vi "Compiled.Get Counter And Protection Frames.vi"(8 "error in (no error)":errorcluster, 9 "Frames per type":T10[](array[typedef]) {"Frame Settings"."Transmit Trigger Ref" format="%.0x"; "Frame Settings"."Disable Transmission Ref" format="%.0x"; "Frame Refs" format="%.0x"}, 10 "GUIDs":T9, 11 "XNET Cluster":refnum<k21>) -> (0 "error out":errorcluster, 1 "Counters and Protection Refs":T1[](array[typedef]) format="%.0x", 2 "Signals Refs":T1[](array[typedef]) format="%.0x", 3 "Frames":T2[](array[typedef]) {"Protection Configurations"."CRC Channels"."Data Type" items=["Signed", "Unsigned", "IEEE Float"]})   [LabVIEW 2015, in "Protection and Counter Support System Explorer.lvlib"]
uses:
  Protection and Counter Support System Explorer.lvlib
  Types/Export Frames List and Type.ctl
  Shared/Types/Exported Frame Type.ctl
  <vilib>/NI Veristand/Custom Device API/Custom Device Item Ref.ctl
  Types/Exported Frame Settings.ctl
  Shared/Types/Exported Event Trigger Type.ctl
  Types/Export Frame GUIDs List.ctl
  Shared/Types/Exported Frame Settings.ctl
  Shared/Types/Exported Protection Settings.ctl
  Shared/Types/Protection Type.ctl
  Shared/Types/XNET Signal Configuration.ctl
  Shared/Types/Exported Counter Settings.ctl
  <vilib>/NI Veristand/Custom Device Tools/Custom Device Utility Library/NI VeriStand - Search for All Items by GUID.vi
  Shared/Protection and Counter Support Shared.lvlib
  <vilib>/NI VeriStand/Custom Device API/Custom Device API.lvlib
  <resource>/objmgr/xnet.rc
  <vilib>/NI VeriStand/Custom Device Tools/Custom Device Utility Library/Custom Device Utility Library.lvlib
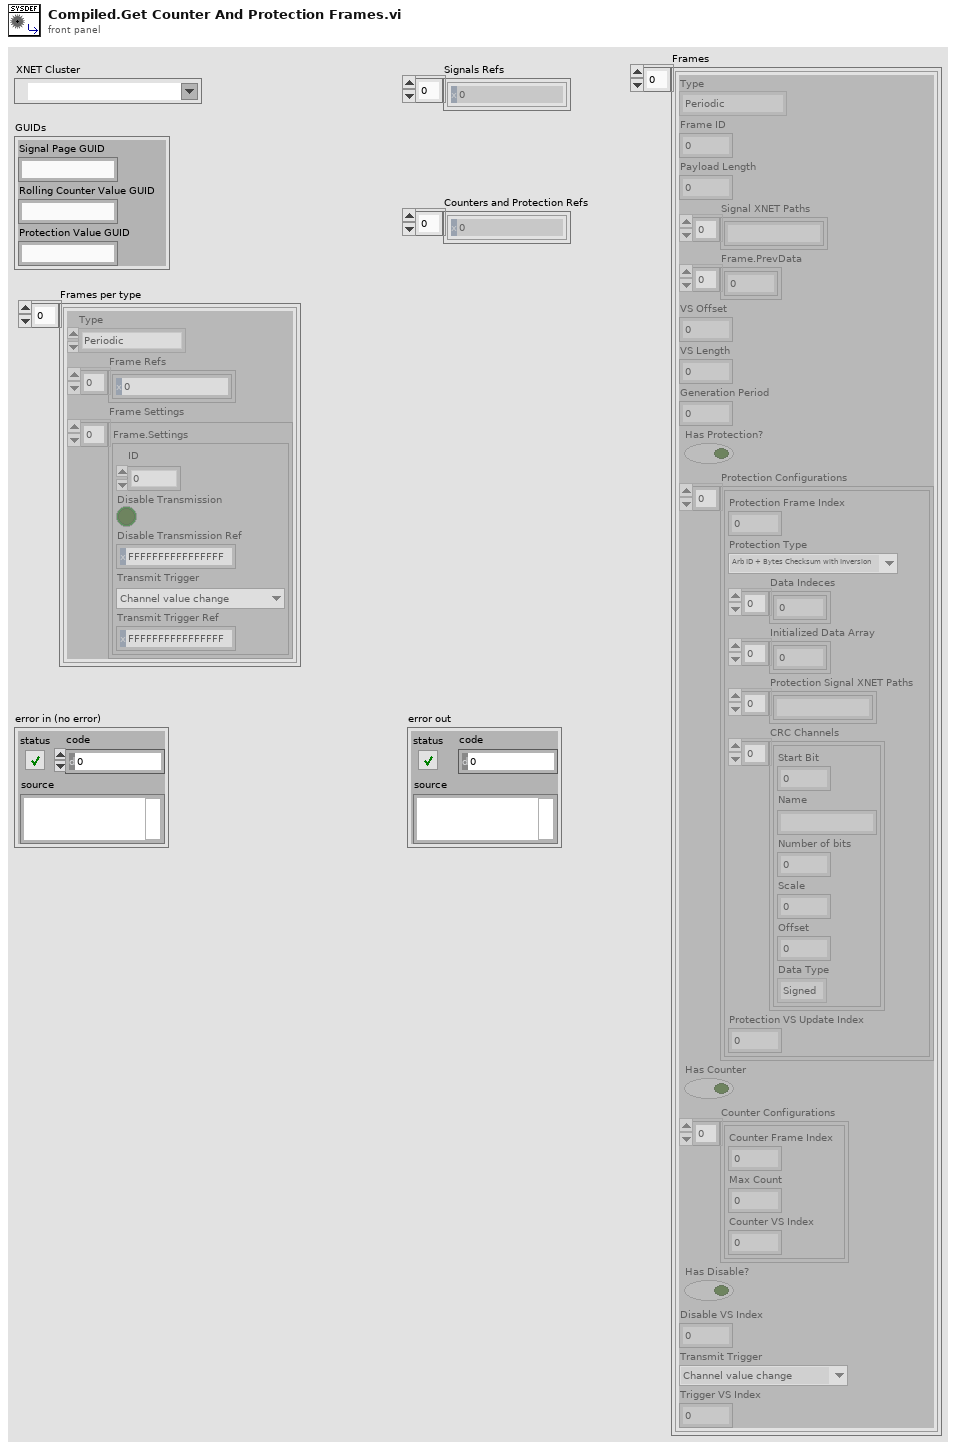
[diagram p1: front panel]
types:
  T1 = typedef "Custom Device API.lvlib/Custom Device Item Ref.ctl" = u64
  T2 = typedef "Protection and Counter Support Shared.lvlib/Exported Frame Settings.ctl" = cluster{"Type":T3, "Frame ID":u32, "Payload Length":u32, "Signal XNET Paths":string[], "Frame.PrevData":dbl[], "VS Offset":i32, "VS Length":i32, "Generation Period":u32, "Has Protection?":bool, "Protection Configurations":T4[], "Has Counter":bool, "Counter Configurations":T7[], "Has Disable?":bool, "Disable VS Index":i32, "Transmit Trigger":T8, "Trigger VS Index":i32}
  T3 = typedef "Protection and Counter Support Shared.lvlib/Exported Frame Type.ctl" = enum16{"Periodic", "Event", "Periodic/Event"}
  T4 = typedef "Protection and Counter Support Shared.lvlib/Exported Protection Settings.ctl" = cluster{"Protection Frame Index":i32, "Protection Type":T5, "Data Indeces":i32[], "Initialized Data Array":dbl[], "Protection Signal XNET Paths":string[], "CRC Channels":T6[], "Protection VS Update Index":i32}
  T5 = typedef "Protection and Counter Support Shared.lvlib/Protection Type.ctl" = enum16{"Arb ID + Bytes Checksum with Inversion", "Arb ID + Bytes CRC with Inversion", "Reversed Raw Signal Checksum with Inversion"}
  T6 = typedef "Protection and Counter Support Shared.lvlib/XNET Signal Configuration.ctl" = cluster{"Start Bit":i32, "Name":string, "Number of bits":i32, "Scale":dbl, "Offset":dbl, "Data Type":u32}
  T7 = typedef "Protection and Counter Support Shared.lvlib/Exported Counter Settings.ctl" = cluster{"Counter Frame Index":i32, "Max Count":dbl, "Counter VS Index":i32}
  T8 = typedef "Protection and Counter Support Shared.lvlib/Exported Event Trigger Type.ctl" = enum16{"Channel value change", "Trigger channel (not zero)", "Channel value change or trigger channel (not zero)", "Trigger channel (any value change)", "Channel value change or trigger channel (any value change)"}
  T9 = typedef "Protection and Counter Support System Explorer.lvlib/Export Frame GUIDs List.ctl" = cluster{"Signal Page GUID":string, "Rolling Counter Value GUID":string, "Protection Value GUID":string}
  T10 = typedef "Protection and Counter Support System Explorer.lvlib/Export Frames List and Type.ctl" = cluster{"Type":T3, "Frame Refs":T1[], "Frame Settings":T11[]}
  T11 = typedef "Protection and Counter Support System Explorer.lvlib/Exported Frame Settings.ctl" = cluster{"ID":u32, "Disable Transmission":bool, "Disable Transmission Ref":T1, "Transmit Trigger":T8, "Transmit Trigger Ref":T1}
  T12 = typedef "Custom Device API.lvlib/Custom Device Item Info.ctl" = cluster{"Name":string, "Is Channel":bool, "GUID":string, "Is Waveform":bool}
  T13 = typedef "Protection and Counter Support System Explorer.lvlib/Protection Signal Settings.ctl" = cluster{"Input Channels":T14[], "Protection Type":T5}
  T14 = typedef "Protection and Counter Support System Explorer.lvlib/Protection Signal Linked Channel.ctl" = cluster{"Node Ref":T1}
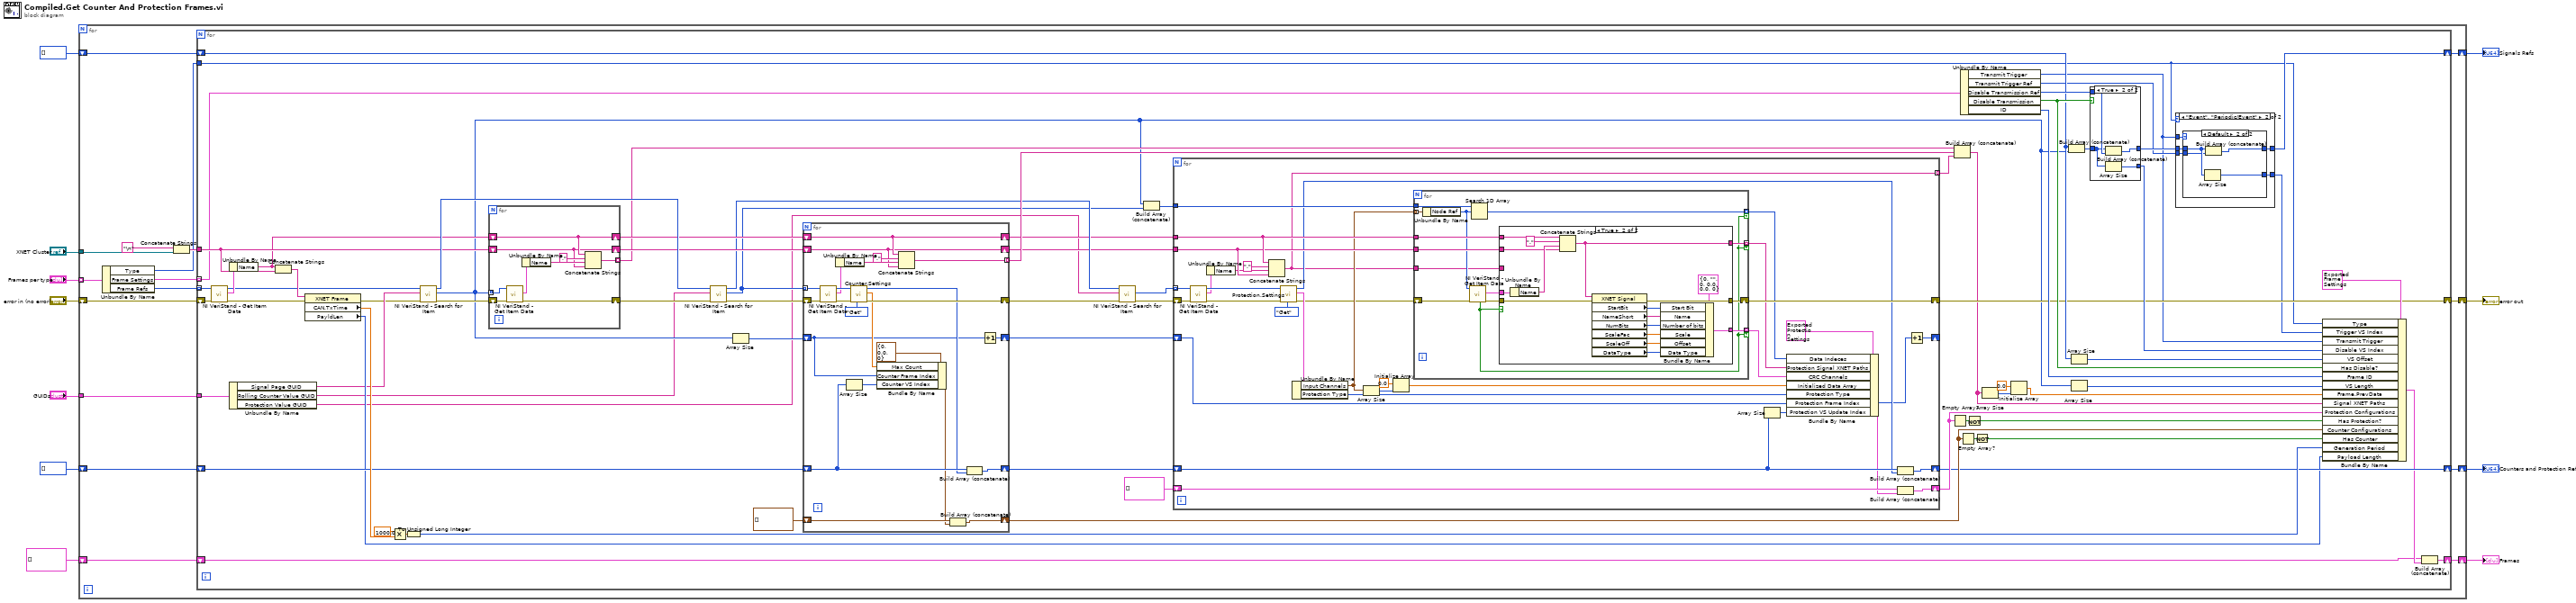
[diagram p0: block diagram]
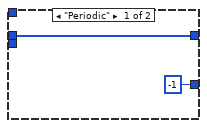
[diagram p2: hidden frame]
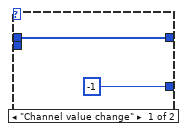
[diagram p3: hidden frame]
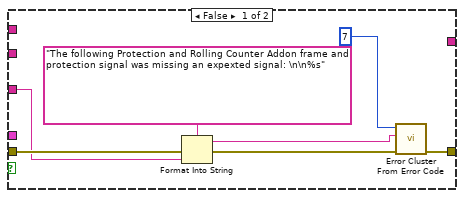
[diagram p4: hidden frame]
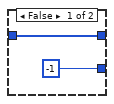
[diagram p5: hidden frame]
diagram:
  n1 = for {
    tunnel: "XNET Cluster" -> [w27]
    shift-right: [w22] -> w4
    shift-left: "error in (no error)" -> [w16]
    shift-right: [w21] -> w5
    shift-left: T2[] [] -> [w20]
    shift-right: [w24] -> w2
    shift-left: T1[] [] -> [w19]
    shift-right: [w23] -> w3
    shift-left: T1[] [] -> [w18]
    tunnel: "GUIDs" -> [w17]
    tunnel: "Frames per type" -> [w15] mode=indexing
    n2 = Unbundle By Name(w15) -> ("Type"=w14:T3, "Frame Settings"=w12:T11[], "Frame Refs"=w13:T1[])
    n3 = Concatenate Strings("\n", w27) -> (w25:string)
    n4 = for {
      tunnel: w13 -> [w83] mode=indexing
      shift-right: [w52] -> w22
      shift-left: w16 -> [w84]
      shift-right: [w95] -> w24
      shift-left: w19 -> [w93]
      tunnel: w25 -> [w68]
      shift-right: [w46] -> w23
      shift-left: w18 -> [w74]
      shift-right: [w37] -> w21
      shift-left: w20 -> [w36]
      tunnel: w14 -> [w35]
      tunnel: w17 -> [w34]
      tunnel: w12 -> [w30] mode=indexing
      n5 = call <vilib>:"NI VeriStand - Get Item Data.vi"("error in (no error)"=w84, "Item Ref in"=w83) -> ("error out"=w80:errorcluster, "Item Info"=w82:T12, "Item Ref out"=w28:T1)  [unwired: 6 in, 1 out]
      n6 = Unbundle By Name(w34) -> ("Signal Page GUID"=w33:string, "Rolling Counter Value GUID"=w32:string, "Protection Value GUID"=w31:string)
      n7 = Unbundle By Name(w82) -> ("Name"=w67:string)
      n8 = Concatenate Strings(w67, w68) -> (w81:string)
      n9 = property class="XNET Frame"(reference=w81, error in=w80) -> (error out=w29:errorcluster, "CAN.TxTime"=w78:dbl, "PayldLen"=w42:u32)  [unwired: 1 out]
      n10 = Multiply(x=1000.0 ("y"), y=w78) -> (x*y=w79:dbl)
      n11 = To Unsigned Long Integer(number=w79) -> (unsigned 32bit integer=w76:u32)
      n12 = call-poly <vilib>:"NI VeriStand - Search for Item.vi"("error in"=w29, "Item GUID"=w33, "Section Ref in"=w28) -> ("error out"=w70:errorcluster, "Item Refs"=w44:T1[], "Section Ref out"=w73:T1)  [unwired: 5 in, 1 out]
      n13 = for {
        tunnel: w44 -> [w192] mode=indexing
        shift-right: [w186] -> w69
        shift-left: w70 -> [w191]
        tunnel: [w188] -> w64 mode=indexing
        shift-right: [w185] -> w66
        shift-left: w67 -> [w185]
        shift-right: [w184] -> w65
        shift-left: w68 -> [w184]
        n14 = call <vilib>:"NI VeriStand - Get Item Data.vi"("error in (no error)"=w191, "Item Ref in"=w192) -> ("error out"=w186:errorcluster, "Item Info"=w187:T12)  [unwired: 6 in, 2 out]
        n15 = Unbundle By Name(w187) -> ("Name"=w189:string)
        n16 = Concatenate Strings(w185, "." ("string"), w189, w184) -> (w188:string)
      }
      n17 = call-poly <vilib>:"NI VeriStand - Search for Item.vi"("error in"=w69, "Item GUID"=w32, "Section Ref in"=w73) -> ("error out"=w72:errorcluster, "Item Refs"=w43:T1[], "Section Ref out"=w61:T1)  [unwired: 5 in, 1 out]
      n18 = Array Size(array=w44) -> (size(s)=w71:i32)
      n19 = for {
        tunnel: w43 -> [w215] mode=indexing
        shift-right: [w209] -> w62
        shift-left: w72 -> [w214]
        shift-right: [w211] -> w85
        shift-left: T7[] [] -> [w210]
        tunnel: [w206] -> w63 mode=indexing
        shift-right: [w203] -> w47
        shift-left: w74 -> [w204]
        shift-right: [w196] -> w57
        shift-left: w71 -> [w197]
        shift-right: [w195] -> w55
        shift-left: w66 -> [w195]
        shift-right: [w194] -> w56
        shift-left: w65 -> [w194]
        n20 = call <vilib>:"NI VeriStand - Get Item Data.vi"("error in (no error)"=w214, "Item Ref in"=w215) -> ("error out"=w212:errorcluster, "Item Info"=w205:T12, "Item Ref out"=w213:T1)  [unwired: 6 in, 1 out]
        n21 = Unbundle By Name(w205) -> ("Name"=w207:string)
        n22 = Array Size(array=w204) -> (size(s)=w198:i32)
        n23 = call "Counter.Settings.vi"("Action"=enum8{"Get", "Set"}."Get", "error in"=w212, "Parent Ref"=w213) -> ("error out"=w209:errorcluster, "Max Count"=w202:dbl, "Parent Ref Out"=w199:T1)  [unwired: 6 in]
        n24 = Bundle By Name(cluster=T7 {"Counter Frame Index"=0, "Max Count"=0.0, "Counter VS Index"=0} ("Cluster"), "Max Count"=w202, "Counter Frame Index"=w197, "Counter VS Index"=w198) -> (w201:T7)
        n25 = Concatenate Strings(w195, "." ("string"), w207, w194) -> (w206:string)
        n26 = Build Array (concatenate)(w210, w201) -> (w211:T7[])
        n27 = Build Array (concatenate)(w204, w199) -> (w203:T1[])
        n28 = Increment(x=w197) -> (x+1=w196:i32)
      }
      n29 = call-poly <vilib>:"NI VeriStand - Search for Item.vi"("error in"=w62, "Item GUID"=w31, "Section Ref in"=w61) -> ("error out"=w60:errorcluster, "Item Refs"=w59:T1[])  [unwired: 5 in, 2 out]
      n30 = Build Array (concatenate)(w44, w43) -> (w45:T1[])
      n31 = for {
        tunnel: w59 -> [w146] mode=indexing
        shift-right: [w139] -> w52
        shift-left: w60 -> [w145]
        shift-right: [w140] -> w53
        shift-left: T4[] [] -> [w142]
        tunnel: w45 -> [w141]
        tunnel: w55 -> [w137]
        tunnel: [w115] -> w54 mode=indexing
        shift-right: [w133] -> w46
        shift-left: w47 -> [w134]
        shift-right: [w117] -> _
        shift-left: w57 -> [w118]
        tunnel: w56 -> [w136]
        n32 = call <vilib>:"NI VeriStand - Get Item Data.vi"("error in (no error)"=w145, "Item Ref in"=w146) -> ("error out"=w143:errorcluster, "Item Info"=w135:T12, "Item Ref out"=w144:T1)  [unwired: 6 in, 1 out]
        n33 = Unbundle By Name(w135) -> ("Name"=w116:string)
        n34 = Concatenate Strings(w137, "." ("string"), w116, w136) -> (w115:string)
        n35 = call "Protection.Settings.vi"("Action"=enum8{"Get", "Set"}."Get", "error in"=w143, "Parent Ref"=w144) -> ("error out"=w123:errorcluster, "Selected Channels"=w132:T13, "Parent Ref Out"=w119:T1)  [unwired: 6 in]
        n36 = Unbundle By Name(w132) -> ("Input Channels"=w129:T14[], "Protection Type"=w131:T5)
        n37 = Array Size(array=w129) -> (size(s)=w128:i32)
        n38 = Initialize Array(0.0 ("element"), w128) -> (w126:dbl[])
        n39 = for {
          tunnel: w141 -> [w150]
          tunnel: w129 -> [w160] mode=indexing
          tunnel: [w159] -> w130 mode=indexing if=w148
          shift-right: [w153] -> w139
          shift-left: w123 -> [w158]
          tunnel: w137 -> [w156]
          tunnel: w136 -> [w155]
          tunnel: [w151] -> w122 mode=indexing if=w148
          tunnel: [w152] -> w124 mode=indexing if=w148
          tunnel: w115 -> [w147]
          n40 = Unbundle By Name(w160) -> ("Node Ref"=w149:T1)
          n41 = call <vilib>:"NI VeriStand - Get Item Data.vi"("error in (no error)"=w158, "Item Ref in"=w149) -> ("error out"=w154:errorcluster, "Item Info"=w157:T12, "Found"=w148:bool)  [unwired: 6 in, 1 out]
          n42 = Search 1D Array(1D array=w150, element=w149) -> (index of element=w159:i32)  [unwired: 1 in]
          n43 = case shown="True" w148 {
            tunnel: w157 -> [_ w183]
            tunnel: w156 -> [_ w180]
            tunnel: w155 -> [_ w179]
            tunnel: w154 -> [w165 w178]
            tunnel: [w167 w177] -> w153
            tunnel: [_ w169] -> w152
            tunnel: [_ w168] -> w151
            tunnel: w147 -> [w162 _]
            frame False {
              n44 = Format Into String(format string="The following Protection and Rolling Counter Addon frame and protection signal was missing an expexted signal: \n\n%s" ("error message (\"\")"), error in=w165, w162) -> (resulting string=w161:string, error out=w164:errorcluster)  [unwired: 1 in]
              n45 = call <vilib>:"Error Cluster From Error Code.vi"("error in (no error)"=w164, "error message (\"\")"=w161, "error code (0)"=7) -> ("error out"=w167:errorcluster)  [unwired: 6 in]
            }
            frame True {
              n46 = Unbundle By Name(w183) -> ("Name"=w181:string)
              n47 = Concatenate Strings(w180, "." ("string"), w181, w179) -> (w168:string)
              n48 = property class="XNET Signal"(reference=w168, error in=w178) -> (error out=w177:errorcluster, "StartBit"=w170:u32, "NameShort"=w171:string, "NumBits"=w172:u32, "ScaleFac"=w173:dbl, "ScaleOff"=w174:dbl, "DataType"=w175:u32)  [unwired: 1 out]
              n49 = Bundle By Name(cluster=T6 {"Start Bit"=0, "Name"="", "Number of bits"=0, "Scale"=0.0, "Offset"=0.0, "Data Type"=0} ("MonitoredChannelSettings"), "Start Bit"=w170, "Name"=w171, "Number of bits"=w172, "Scale"=w173, "Offset"=w174, "Data Type"=w175) -> (w169:T6)
            }
          }
        }
        n50 = Array Size(array=w134) -> (size(s)=w120:i32)
        n51 = Bundle By Name(cluster=T4 {"Protection Frame Index"=0, "Protection Type"=enum."Arb ID + Bytes Checksum with Inversion", "Data Indeces"=[], "Initialized Data Array"=[], "Protection Signal XNET Paths"=[], "CRC Channels"=[], "Protection VS Update Index"=0} ("Cluster"), "Data Indeces"=w130, "Protection Signal XNET Paths"=w122, "CRC Channels"=w124, "Initialized Data Array"=w126, "Protection Type"=w131, "Protection Frame Index"=w118, "Protection VS Update Index"=w120) -> (w125:T4)
        n52 = Build Array (concatenate)(w134, w119) -> (w133:T1[])
        n53 = Build Array (concatenate)(w142, w125) -> (w140:T4[])
        n54 = Increment(x=w118) -> (x+1=w117:i32)
      }
      n55 = Empty Array?(array=w53) -> (empty?=w87:bool)
      n56 = Build Array (concatenate)(w64, w63, w54) -> (w51:string[])
      n57 = Unbundle By Name(w30) -> ("Transmit Trigger"=w40:T8, "Transmit Trigger Ref"=w41:T1, "Disable Transmission Ref"=w97:T1, "Disable Transmission"=w98:bool, "ID"=w99:u32)
      n58 = Empty Array?(array=w85) -> (empty?=w89:bool)
      n59 = Not(x=w87) -> (.not. x?=w86:bool)
      n60 = Not(x=w89) -> (.not. x?=w88:bool)
      n61 = Array Size(array=w51) -> (size(s)=w49:i32)
      n62 = Initialize Array(0.0 ("element"), w49) -> (w48:dbl[])
      n63 = Build Array (concatenate)(w93, w44) -> (w94:T1[])
      n64 = Array Size(array=w93) -> (size(s)=w92:i32)
      n65 = Array Size(array=w44) -> (size(s)=w75:i32)
      n66 = case shown="True" w98 {
        tunnel: w94 -> [w217 w219]
        tunnel: [w217 w221] -> w96
        tunnel: w97 -> [_ w220]
        tunnel: [-1 w218] -> w91
        frame False {
        }
        frame True {
          n67 = Build Array (concatenate)(w219, w220) -> (w221:T1[])
          n68 = Array Size(array=w219) -> (size(s)=w218:i32)
        }
      }
      n69 = case shown="\"Event\", \"Periodic/Event\"" w35 {
        tunnel: w96 -> [w102 w107]
        tunnel: [w102 w106] -> w95
        tunnel: w41 -> [_ w105]
        tunnel: w40 -> [_ w104]
        tunnel: [-1 w103] -> w39
        frame "Periodic" {
        }
        frame "Event", "Periodic/Event" {
          n70 = case shown="Default" w104 {
            tunnel: w107 -> [w109 w112]
            tunnel: [w109 w113] -> w106
            tunnel: [-1 w111] -> w103
            tunnel: w105 -> [_ w110]
            frame "Channel value change" {
            }
            frame Default {
              n71 = Array Size(array=w112) -> (size(s)=w111:i32)
              n72 = Build Array (concatenate)(w112, w110) -> (w113:T1[])
            }
          }
        }
      }
      n73 = Bundle By Name(cluster=T2 {"Type"=enum."Periodic", "Frame ID"=0, "Payload Length"=0, "Signal XNET Paths"=[], "Frame.PrevData"=[], "VS Offset"=0, "VS Length"=0, "Generation Period"=0, "Has Protection?"=FALSE, "Protection Configurations"=[], "Has Counter"=FALSE, "Counter Configurations"=[], "Has Disable?"=FALSE, "Disable VS Index"=0, "Transmit Trigger"=enum."Channel value change", "Trigger VS Index"=0} ("Frame Settings"), "Type"=w35, "Trigger VS Index"=w39, "Transmit Trigger"=w40, "Disable VS Index"=w91, "VS Offset"=w92, "Has Disable?"=w98, "Frame ID"=w99, "VS Length"=w75, "Frame.PrevData"=w48, "Signal XNET Paths"=w51, "Protection Configurations"=w53, "Has Protection?"=w86, "Counter Configurations"=w85, "Has Counter"=w88, "Generation Period"=w76, "Payload Length"=w42) -> (w38:T2)
      n74 = Build Array (concatenate)(w36, w38) -> (w37:T2[])
    }
  }
  "Frames" <- w5
  "error out" <- w4
  "Counters and Protection Refs" <- w3
  "Signals Refs" <- w2
